vi "Read Photodiodes.vi"(0 "Sample Rate (Hz)":dbl=1000000.0 format="%0.2f", 1 "Time to sample (seconds)":dbl=2.0, 2 "Buffer size (samples per channel)":u32=2000000, 3 "Current test directory":path) -> ()   [LabVIEW 2018]
uses:
  <vilib>/DAQmx/read.llb/DAQmx Read (Analog 1D Wfm NChan NSamp).vi
  <vilib>/DAQmx/create/channels.llb/DAQmx Create Channel (AI-Voltage-Basic).vi
  <vilib>/DAQmx/configure/timing.llb/DAQmx Timing (Sample Clock).vi
  <vilib>/DAQmx/miscellaneous.llb/DAQmx Fill In Error Info.vi
panel:
  out "data":waveform(dbl)[](graph) caption="Diode Data"
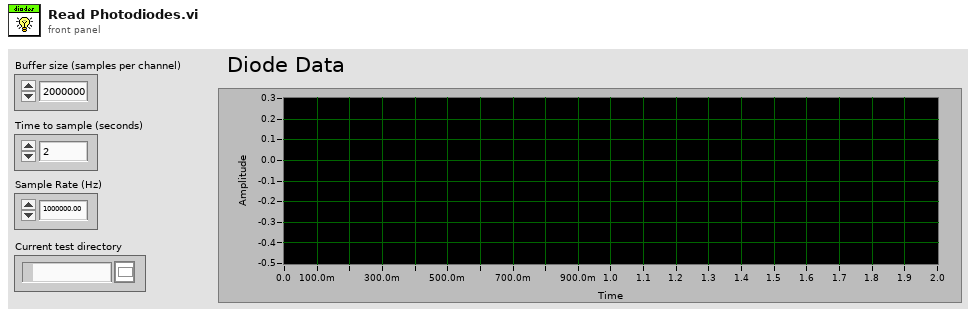
[diagram p1: front panel]
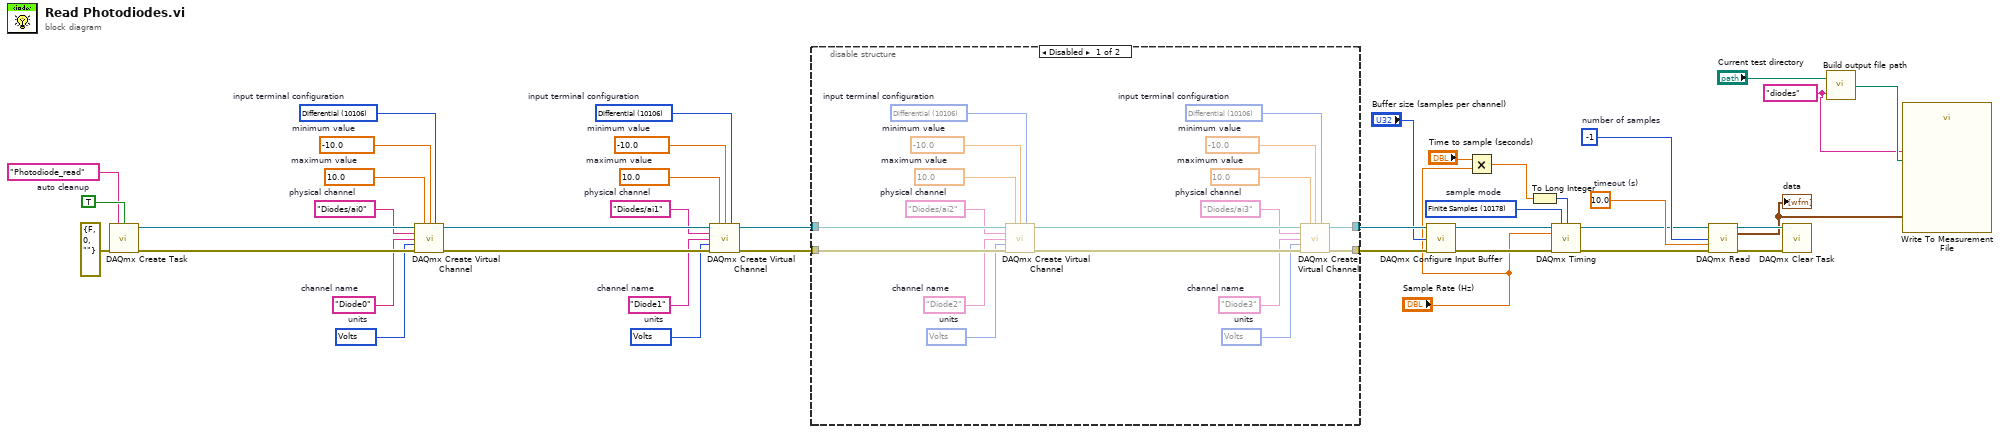
[diagram p0: block diagram]
diagram:
  w2 = "diodes" ("Measurement type")
  w11 = 10106 items=["default"=-1, "RSE"=10083, "NRSE"=10078, "Differential"=10106, "Pseudodifferential"=12529]  # input terminal configuration
  w12 = 10348 items=["Volts"=10348, "From Custom Scale"=10065]  # units
  w13 = "Diode1"  # channel name
  w15 = -10.0  # minimum value
  w16 = 10.0  # maximum value
  w17 = "Diodes/ai1"  # physical channel
  w19 = 10106 items=["default"=-1, "RSE"=10083, "NRSE"=10078, "Differential"=10106, "Pseudodifferential"=12529]  # input terminal configuration
  w20 = 10348 items=["Volts"=10348, "From Custom Scale"=10065]  # units
  w21 = "Diode0"  # channel name
  w23 = -10.0  # minimum value
  w24 = 10.0  # maximum value
  w25 = "Diodes/ai0"  # physical channel
  w27 = 10178 items=["Finite Samples"=10178, "Continuous Samples"=10123, "Hardware Timed Single Point"=12522]  # sample mode
  w36 = TRUE  # auto cleanup
  w40 = 10.0  # timeout (s)
  w41 = -1  # number of samples
  n1 = call <vilib>:"DAQmx Create Task.vi"("new task name"="Photodiode_read", "auto cleanup"=w36, "error in"=errorcluster {"status"=FALSE, "code"=0, "source"=""}) -> ("task out"=w35:refnum<k21>, "error out"=w37:errorcluster)  [unwired: 11 in]
  n2 = call-poly <vilib>:"DAQmx Create Virtual Channel.vi"("task in"=w35, "maximum value"=w24, "minimum value"=w23, "input terminal configuration"=w19, "physical channels"=w25, "name to assign"=w21, "units"=w20, "error in"=w37) -> ("task out"=w18:refnum<k21>, "error out"=w22:errorcluster)  [unwired: 6 in]
  n3 = call-poly <vilib>:"DAQmx Create Virtual Channel.vi"("task in"=w18, "maximum value"=w16, "minimum value"=w15, "input terminal configuration"=w11, "physical channels"=w17, "name to assign"=w13, "units"=w12, "error in"=w22) -> ("task out"=w10:refnum<k21>, "error out"=w14:errorcluster)  [unwired: 6 in]
  n4 = disable-structure shown="Disabled" {
    disable-tunnel: [w59 w61] -> w31
    disable-tunnel: [w58 w60] -> w30
    disable-tunnel: w14 -> [w57 w60]
    disable-tunnel: w10 -> [w56 w61]
    frame Disabled {
      w42 = 10106 items=["default"=-1, "RSE"=10083, "NRSE"=10078, "Differential"=10106, "Pseudodifferential"=12529]  # input terminal configuration
      w43 = 10348 items=["Volts"=10348, "From Custom Scale"=10065]  # units
      w44 = "Diode3"  # channel name
      w45 = -10.0  # minimum value
      w46 = 10.0  # maximum value
      w47 = "Diodes/ai3"  # physical channel
      w48 = 10106 items=["default"=-1, "RSE"=10083, "NRSE"=10078, "Differential"=10106, "Pseudodifferential"=12529]  # input terminal configuration
      w49 = 10348 items=["Volts"=10348, "From Custom Scale"=10065]  # units
      w50 = "Diode2"  # channel name
      w51 = -10.0  # minimum value
      w52 = 10.0  # maximum value
      w53 = "Diodes/ai2"  # physical channel
      n5 = call-poly <vilib>:"DAQmx Create Virtual Channel.vi"("task in"=w56, "maximum value"=w52, "minimum value"=w51, "input terminal configuration"=w48, "physical channels"=w53, "name to assign"=w50, "units"=w49, "error in"=w57) -> ("task out"=w54:refnum<k21>, "error out"=w55:errorcluster)  [unwired: 6 in]
      n6 = call-poly <vilib>:"DAQmx Create Virtual Channel.vi"("task in"=w54, "maximum value"=w46, "minimum value"=w45, "input terminal configuration"=w42, "physical channels"=w47, "name to assign"=w44, "units"=w43, "error in"=w55) -> ("task out"=w59:refnum<k21>, "error out"=w58:errorcluster)  [unwired: 6 in]
    }
    frame Enabled {
    }
  }
  n7 = call <vilib>:"DAQmx Configure Input Buffer.vi"("task/channels in"=w31, "buffer size (in samples per channel)"="Buffer size (samples per channel)", "error in"=w30) -> ("task out"=w26:refnum<k21>, "error out"=w29:errorcluster)  [unwired: 11 in]
  n8 = Multiply(x="Time to sample (seconds)", y="Sample Rate (Hz)") -> (x*y=w6:dbl)
  n9 = To Long Integer(number=w6) -> (32bit integer=w5:i32)
  n10 = call-poly <vilib>:"DAQmx Timing.vi"("task/channels in"=w26, "sample mode"=w27, "samples per channel"=w5, "rate"="Sample Rate (Hz)", "error in"=w29) -> ("task out"=w34:refnum<k21>, "error out"=w33:errorcluster)  [unwired: 9 in]
  n11 = call-poly <vilib>:"DAQmx Read.vi"("task/channels in"=w34, "number of samples per channel"=w41, "timeout"=w40, "error in"=w33) -> ("task out"=w38:refnum<k21>, "data"=w4:waveform(dbl)[], "error out"=w39:errorcluster)  [unwired: 9 in]
  "data" <- w4
  n12 = call <vilib>:"DAQmx Clear Task.vi"("task in"=w38, "error in"=w39) -> ()  [unwired: 13 in, 1 out]
  n13 = call "Build output file path.vi"("Measurement type"=w2, "Current test directory"="Current test directory") -> ("File path"=w3:path)
  n14 = call "Write To Measurement File"("Signals"=w4, "Filename"=w3, "Comment"=w2) -> ()  [unwired: 14 in, 3 out]
